vi "update table.vi"(5 "Sort By...":T3 items=["RIO device", "resource", "input type", "datatype", "reserver"], 6 "Filter in":refnum<class "Filter.lvclass">, 7 "selected values":bool[](array[boolean]), 8 "error in (no error)":errorcluster, 9 "Show":T1, 10 "MulticolumnListbox in":refnum<vi>, 11 "Item Ref in":T2 format="%.0x") -> (0 "error out":errorcluster, 2 "max string length in columns":i32[](array[numeric]), 3 "resource entries":T4[](array[typedef]) {"FPGA CD Ref" format="%.0x"; "reserver" format="%.0x"})   [LabVIEW 2016, in "FPGA Resource Manager.lvlib"]
uses:
  FPGA Resource Manager.lvlib
  resource info.ctl
  <vilib>/NI Veristand/Custom Device API/Custom Device Item Ref.ctl
  viz_type.ctl
  viz_show.ctl
  Filters/Filter Parent/Filter.lvclass
  global constants.vi
  <vilib>/NI VeriStand/Custom Device API/Custom Device API.lvlib
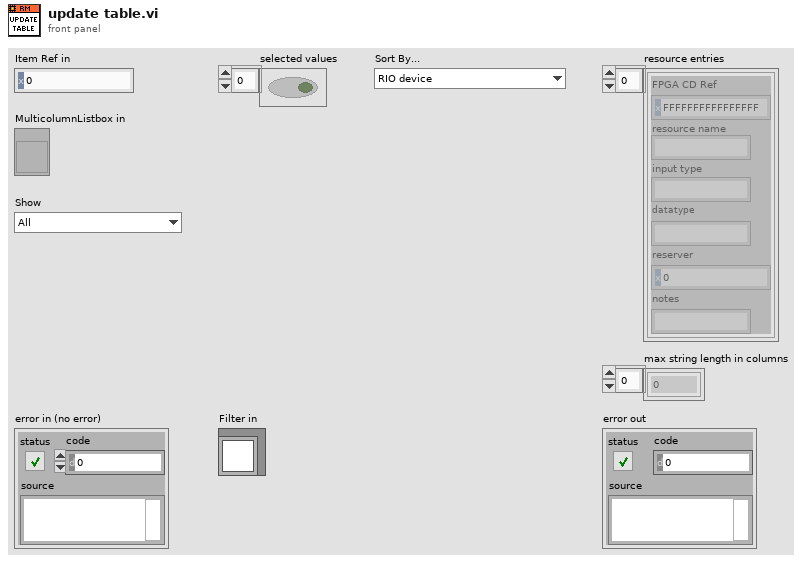
[diagram p1: front panel]
types:
  T1 = typedef "FPGA Resource Manager.lvlib/viz_show.ctl" = enum16{"All", "Mapped", "Unmapped"}
  T2 = typedef "Custom Device API.lvlib/Custom Device Item Ref.ctl" = u64
  T3 = typedef "FPGA Resource Manager.lvlib/viz_type.ctl" = u16
  T4 = typedef "FPGA Resource Manager.lvlib/resource info.ctl" = cluster{"FPGA CD Ref":T2, "resource name":string, "input type":string, "datatype":string, "reserver":T2, "notes":string}
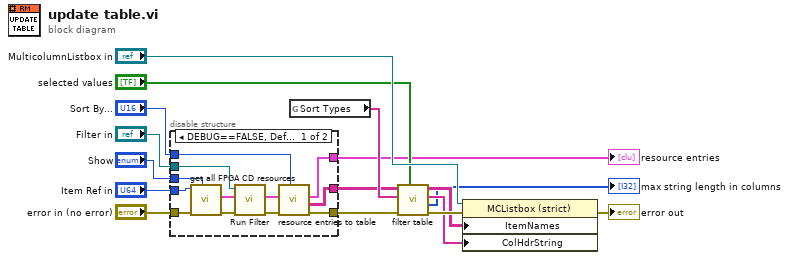
[diagram p0: block diagram]
diagram:
  n1 = disable-structure shown="DEBUG==FALSE, Default" {
    disable-tunnel: "error in (no error)" -> [w28 w29]
    disable-tunnel: "Item Ref in" -> [w27 _]
    disable-tunnel: [w25 w29] -> w15
    disable-tunnel: [w17 _] -> w2
    disable-tunnel: "Show" -> [w24 _]
    disable-tunnel: [w18 _] -> w5
    disable-tunnel: "Sort By..." -> [w23 _]
    disable-tunnel: "Filter in" -> [w22 _]
    frame condition #0 (active) {
      n2 = call "get all FPGA CD resources.vi"("Show"=w24, "error in (no error)"=w28, "Item Ref in"=w27) -> ("error out"=w21:errorcluster, "resource entries"=w26:T4[])  [unwired: 6 in, 1 out]
      n3 = call-dynamic "Run Filter.vi"("error in (no error)"=w21, "resource entries in"=w26, "Filter in"=w22) -> ("error out"=w20:errorcluster, "resource entries out"=w19:T4[])  [unwired: 7 in]
      n4 = call "resource entries to table.vi"("Sort Type"=w23, "error in (no error)"=w20, "resource entries"=w19) -> ("error out"=w25:errorcluster, "sorted resource table out"=w18:string[][], "sorted resource entries out"=w17:T4[])  [unwired: 6 in]
    }
    frame condition #1 {
    }
  }
  "resource entries" <- w2
  n5 = global read "global constants.vi" "Sort Types"() -> (w14:string[])
  n6 = call "filter table.vi"("display column?"="selected values", "error in (no error)"=w15, "Sort Types"=w14, "resource table in"=w5) -> ("error out"=w16:errorcluster, "max string length in columns"=→"max string length in columns":i32[], "Headers"=w12:string[], "resource table out"=w13:string[][])  [unwired: 4 in]
  n7 = property on="Property Node" class="MCListbox (strict)"(reference="MulticolumnListbox in", error in=w16, "ItemNames"=w13, "ColHdrString"=w12) -> (error out=→"error out":errorcluster)  [unwired: 1 out]
